vi "Fault Handling.vi"(8 "error in (no error)":errorcluster, 10 "Sequence Context":refnum<k7>, 11 "OPC UA in":refnum<class "OPC UA.lvclass">) -> (0 "error out":errorcluster, 3 "OPC UA out":refnum<class "OPC UA.lvclass">)   [LabVIEW 2019, in "OPC UA.lvlib" / "OPC UA.lvclass"]
uses:
  OPC UA.lvclass
  OPC UA.lvclass/OPC UA.ctl
  <vilib>/addons/TestStand/_TSUtility.llb/TestStand - Set Property Value (String).vi
  <vilib>/addons/TestStand/_TSUtility.llb/TestStand - Set Property Value (Number).vi
panel:
  out "FaultCode":u32
  out "Fault codes":cluster{"Bit":string, "Description":string}[](array[cluster])
  out "Fault":bool
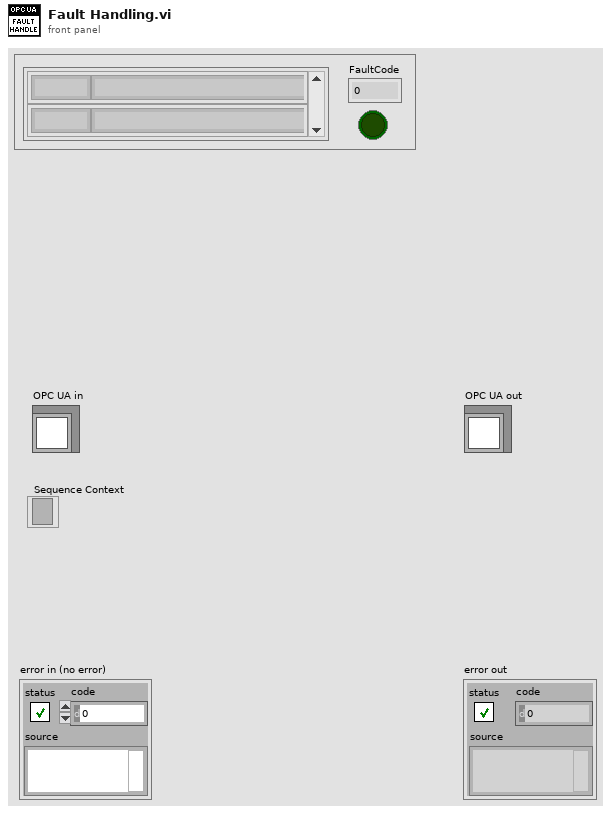
[diagram p1: front panel]
types:
  T1 = typedef "OPC UA.lvlib/OPC UA.lvclass/Tester Rx Dataset.ctl" = cluster{"Start":bool, "NestStatus":bool, "PalletID":u32, "BarcodeData":string, "StepEcho":u32, "Cylinder_1":bool, "Cylinder_2":bool, "Cylinder_3":bool, "Cylinder_4":bool, "Cylinder_5":bool, "ResultsAck":bool, "Reset":bool, "Stop":bool, "FaultCode":u32}
  T2 = typedef "OPC UA.lvlib/OPC UA.lvclass/Tester Tx Dataset.ctl" = cluster{"Fault":bool, "StepNo":u32, "Ready":bool, "HighVoltage":bool, "TestRunning":bool, "ResultsReady":bool, "Results":u32, "ElapsedTime":u32, "Online":bool, "TimeCompleted":i32[], "Timeout":bool, "Heartbeat":bool}
  T3 = enum32{"Invalid", "Standard", "Closed", "Hidden", "Minimized", "Maximized"}
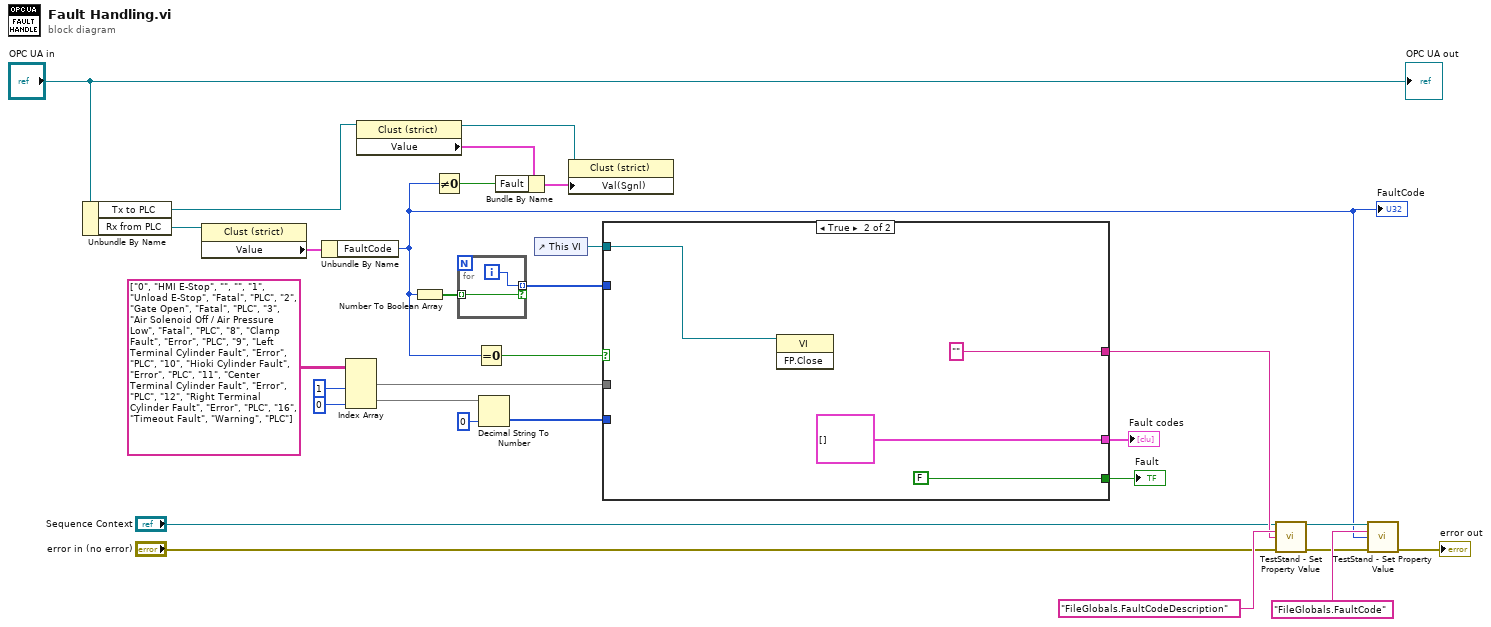
[diagram p0: block diagram]
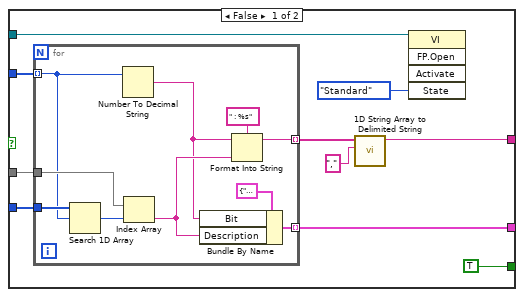
[diagram p2: hidden frame]
diagram:
  n1 = Unbundle By Name("OPC UA in") -> ("Tx to PLC"=w5:refnum<vi>, "Rx from PLC"=w18:refnum<vi>)
  n2 = property class="Clust (strict)"(reference=w18) -> ("Value"=w17:T1)  [unwired: 1 in, 2 out]
  n3 = Unbundle By Name(w17) -> ("FaultCode"=w3:u32)
  "FaultCode" <- w3
  n4 = Index Array(array=string[][] [["0", "HMI E-Stop", "", ""], ["1", "Unload E-Stop", "Fatal", "PLC"], ["2", "Gate Open", "Fatal", "PLC"], ["3", "Air Solenoid Off / Air Pressure Low", "Fatal", "PLC"], ["8", "Clamp Fault", "Error", "PLC"], ["9", "Left Terminal Cylinder Fault", "Error", "PLC"], ["10", "Hioki Cylinder Fault", "Error", "PLC"], ["11", "Center Terminal Cylinder Fault", "Error", "PLC"], ["12", "Right Terminal Cylinder Fault", "Error", "PLC"], ["16", "Timeout Fault", "Warning", "PLC"]], index (col) #1=1 ("disabled index (col)"), index (col) #2=0 ("index (col)")) -> (element #1=w23:string[], element #2=w30:string[])  [unwired: 2 in]
  n5 = property class="Clust (strict)"(reference=w5) -> (reference out=w6:refnum<vi>, "Value"=w8:T2)  [unwired: 1 in, 1 out]
  n6 = Number To Boolean Array(number=w3) -> (Boolean array=w28:bool[])
  n7 = Not Equal To 0?(x=w3) -> (x != 0?=w7:bool)
  n8 = for {
    tunnel: w28 -> [w31] mode=indexing
    tunnel: [w32] -> w25 mode=indexing if=w31
    i -> [w32]
  }
  n9 = Equal To 0?(x=w3) -> (x = 0?=w2:bool)
  n10 = Decimal String To Number(string=w30, default (0L)=0 ("default (0 I32)")) -> (number=w24:i32[])  [unwired: 1 in, 1 out]
  n11 = Bundle By Name(cluster=w8, "Fault"=w7) -> (w9:T2)
  n12 = control-ref of="This VI"() -> (w1:refnum<vi>)
  n13 = property class="Clust (strict)"(reference=w6, "Val(Sgnl)"=w9) -> ()  [unwired: 1 in, 2 out]
  n14 = case shown="True" w2 {
    tunnel: [w38 cluster{"Bit":string, "Description":string}[] []] -> w20
    tunnel: [TRUE FALSE] -> w21
    tunnel: w24 -> [w41 _]
    tunnel: w25 -> [w40 _]
    tunnel: w23 -> [w39 _]
    tunnel: [w36 "" ("delimited string")] -> w14
    tunnel: w1 -> [w33 w53]
    frame False {
      n15 = for {
        tunnel: w40 -> [w48] mode=indexing
        tunnel: w41 -> [w52]
        tunnel: w39 -> [w50]
        tunnel: [w47] -> w38 mode=indexing
        tunnel: [w43] -> w35 mode=indexing
        n16 = Search 1D Array(1D array=w52, element=w48) -> (index of element=w51:i32)  [unwired: 1 in]
        n17 = Number To Decimal String(number=w48) -> (decimal integer string=w44:string)  [unwired: 1 in]
        n18 = Index Array(array=w50, index=w51) -> (element=w45:string)
        n19 = Bundle By Name(cluster=cluster{"Bit":string, "Description":string} {"Bit"="", "Description"=""} ("Fault"), "Bit"=w44, "Description"=w45) -> (w47:cluster{"Bit":string, "Description":string})
        n20 = Format Into String(format string=" : %s", initial string=w44, w45) -> (resulting string=w43:string)  [unwired: 1 in, 1 out]
      }
      n21 = call <vilib>:"1D String Array to Delimited String.vi"("delimiter"=",", "string array"=w35) -> ("delimited string"=w36:string)  [unwired: 9 in]
      n22 = invoke class="VI" method="FP.Open"(reference=w33, "State"=T3."Standard") -> ()  [unwired: 3 in, 5 out]
    }
    frame True {
      n23 = invoke class="VI" method="FP.Close"(reference=w53) -> ()  [unwired: 2 in, 3 out]
    }
  }
  "Fault" <- w21
  "Fault codes" <- w20
  n24 = call-poly <vilib>:"TestStand - Set Property Value.vi"("Sequence Context In"="Sequence Context", "Lookup String"="FileGlobals.FaultCodeDescription", "New Value"=w14, "error in (no error)"="error in (no error)") -> ("Sequence Context Out"=w11:refnum<k7>, "error out"=w12:errorcluster)  [unwired: 10 in]
  n25 = call-poly <vilib>:"TestStand - Set Property Value.vi"("Sequence Context In"=w11, "Lookup String"="FileGlobals.FaultCode", "New Value"=w3, "error in (no error)"=w12) -> ("error out"=→"error out":errorcluster)  [unwired: 10 in, 1 out]
  "OPC UA out" <- "OPC UA in"
